vi "StartVideo End.vi"(8 "error in (no error)":errorcluster, 11 "VLC Variables In in":T1) -> (0 "error out":errorcluster, 3 "VLC Variables In out":T1)   [LabVIEW 2012]
uses:
  Controls-Webcam/VLC Var.ctl
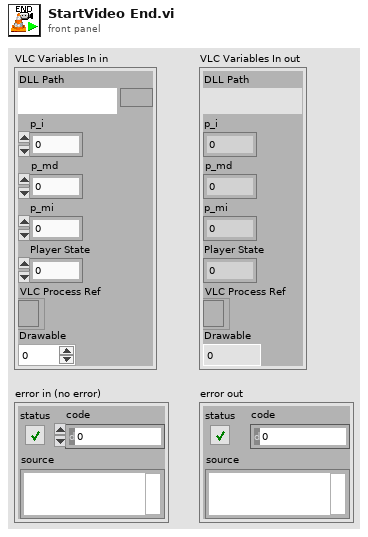
[diagram p1: front panel]
types:
  T1 = typedef "VLC Var.ctl" = cluster{"DLL Path":path, "p_i":i32, "p_md":i32, "p_mi":i32, "Player State":i32, "VLC Process Ref":refnum<k24>, "Drawable":i32}
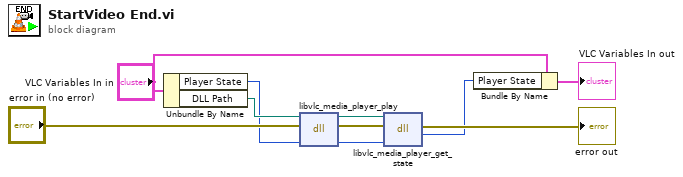
[diagram p0: block diagram]
diagram:
  n1 = Unbundle By Name("VLC Variables In in") -> ("Player State"=w5:i32, "DLL Path"=w10:path)
  n2 = dll-call lib="C:/Program Files (x86)/VideoLAN/VLC/libvlc.dll" fn="libvlc_media_player_play"(path in=w10, error in="error in (no error)", "p_mi"=w5) -> (path out=w4:path, error out=w3:errorcluster, "p_mi"=w2:i32)  [unwired: 2 in]
  n3 = dll-call lib="C:/Program Files/VideoLAN/VLC/libvlc.dll" fn="libvlc_media_player_get_state"(path in=w4, error in=w3, "p_mi"=w2) -> (error out=→"error out":errorcluster, "return type"=w1:i32)  [unwired: 2 in, 1 out]
  n4 = Bundle By Name(cluster="VLC Variables In in", "Player State"=w1) -> (→"VLC Variables In out":T1)
